vi "Update Current Interval Indicator.vi"(4 "Interval idx":u32, 5 "Protocol.Active Interval":T1[](array[typedef])) -> (2 "Protocol.Active Interval":bool[](array[boolean]))   [LabVIEW 2019]
uses:
  Controls/Interval on-off indicator.ctl
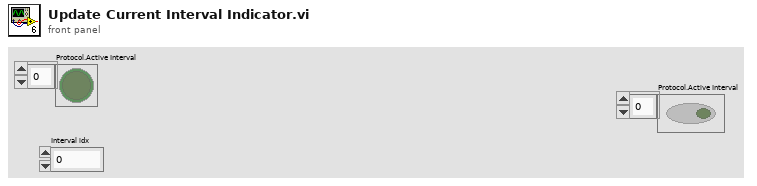
[diagram p1: front panel]
types:
  T1 = typedef "Interval on-off indicator.ctl" = bool
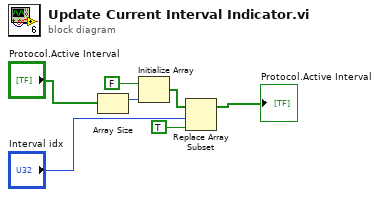
[diagram p0: block diagram]
diagram:
  n1 = Array Size(array="Protocol.Active Interval") -> (size(s)=w4:i32)
  n2 = Initialize Array(FALSE ("element"), w4) -> (w2:bool[])
  n3 = Replace Array Subset(array=w2, new element=TRUE ("new element/subarray"), index="Interval idx") -> (→"Protocol.Active Interval":bool[])
